vi "Mech Calculate Drive Power2.vi"(2 "Reverse":bool, 3 "Deadband (10)":i8=10 min=0 max=100 step=1, 4 "Controller State":T1={"Left X"=0, "Left Y"=0, "Right X"=0, "Right Y"=0, "Button Encoding 9-12"=0, "Button Encoding 1-8"=0, "POV"=-1} {"POV" items=["None"=-1, "POV Up"=0, "POV Up Right"=1, "POV Right"=2, "POV Down Right"=3, "POV Down"=4, "POV Down Left"=5, "POV Left"=6, "POV Up Left"=7]}, 5 "Power Level (50)":i8=50 min=-100 max=100) -> (0 "Right Front Power":i8, 1 "Left Front Power":i8)   [LabVIEW 2012]
doc: "Determines the amount of power to apply to a pair of motors according to the x and y values of a single joystick (Arcade mode) or the y values of each joystick (Tank mode) on a game controller.\nSelect <B>Arcade Steering</B> or <B>Tank Steering</B> from the polymorphic selector on the VI to drive the robot with one joystick or two joysticks respectively.\n\n<B>Inputs</B>\n<B>Reverse</B> specifies, when TRUE, that the motors move in the reverse direction. The default is FALSE.\n<B>Power Level</B> specifies the maximum amount of power to apply to the motor. For example, a value of 50 scales the full range of the joystick to a range of -50 to 50. A negative value drives the motor with the same power as its equivalent positive number but in the opposite direction. You can specify a value between -100 and 100. A value of 0 specifies the motor does not move. The default is 50.\n<B>Controller State</B> specifies the values of the joystick axes and button states of the game controller.\n<B>Deadband</B> specifies the joystick values that the VI treats as zero. When the position of the joystick is within the range you specify, the VI considers the joystick to be at position 0. The default range is -10 to 10.\n\n<B>Outputs</B>\n<B>Left Motor Power</B> returns the amount of power to apply to the left motor. \n<B>Right Motor Power</B> returns the amount of power to apply to the right motor."
uses:
  <vilib>/FTC/FTC ControllerState.ctl
  <vilib>/FTC/FTC POVState.ctl
  <vilib>/NXT/HiTechnic/Calculate Power from Joystick Arcade v2.vi
panel:
  out "Right Rear Power":i8
  out "Left Rear Power":i8
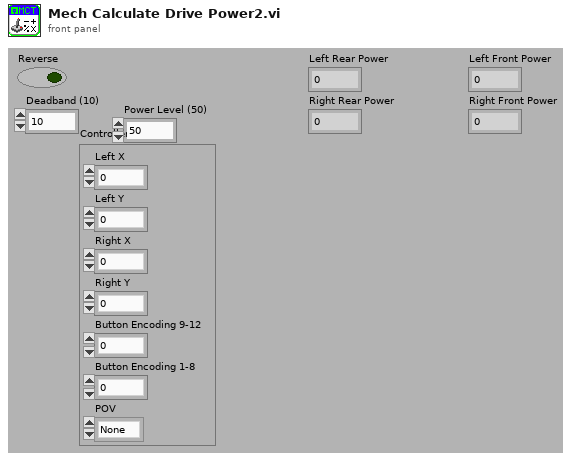
[diagram p1: front panel]
types:
  T1 = typedef "FTC ControllerState.ctl" = cluster{"Left X":i8, "Left Y":i8, "Right X":i8, "Right Y":i8, "Button Encoding 9-12":u8, "Button Encoding 1-8":u8, "POV":T2}
  T2 = typedef "FTC POVState.ctl" = i8
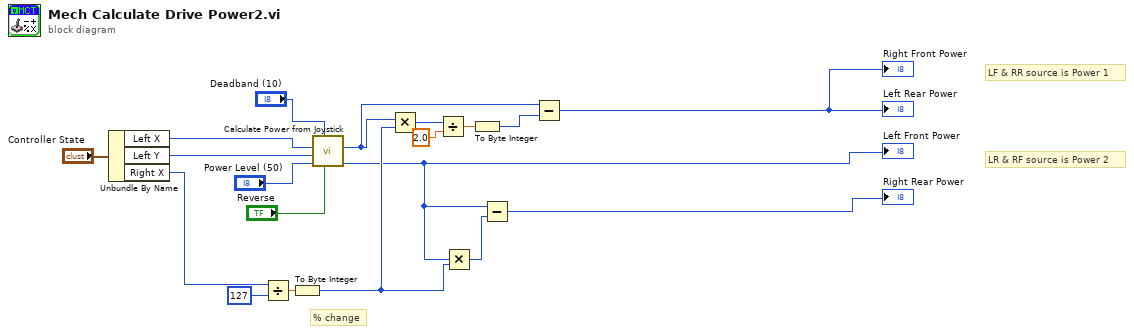
[diagram p0: block diagram]
diagram:
  # "LR & RF source is Power 2"
  # "LF & RR source is Power 1"
  # "% change"
  n1 = Unbundle By Name("Controller State") -> ("Left X"=w18:i8, "Left Y"=w17:i8, "Right X"=w13:i8)
  n2 = Divide(x=w13, y=i8 127) -> (x/y=w11:dbl)
  n3 = To Byte Integer(number=w11) -> (8bit integer=w9:i8)
  n4 = call-poly <vilib>:"Calculate Power from Joystick.vi"("Reverse"="Reverse", "Deadband (10)"="Deadband (10)", "Throttle (50)"="Power Level (50)", "Y Axis"=w17, "X Axis"=w18) -> ("Power 2"=w2:i8, "Power 1"=w4:i8)  [unwired: 4 in, 1 out]
  "Left Front Power" <- w2
  n5 = Multiply(x=w4, y=w9) -> (x*y=w7:i8)
  n6 = Divide(x=w7, y=2.0) -> (x/y=w6:dbl)
  n7 = Multiply(x=w2, y=w9) -> (x*y=w10:i8)
  n8 = To Byte Integer(number=w6) -> (8bit integer=w5:i8)
  n9 = Subtract(x=w2, y=w10) -> (x-y=→"Right Rear Power":i8)
  n10 = Subtract(x=w4, y=w5) -> (x-y=→"Right Front Power" →"Left Rear Power":i8)
